vi "Read Sweep Rate.vi"(8 "error in (no error)":errorcluster, 11 "Power Supply in":refnum<class "Power Supply.lvclass">) -> (0 "error out":errorcluster, 2 "Field sweep rate":dbl[unit], 3 "Power Supply out":refnum<class "Power Supply.lvclass">)   [LabVIEW 2009, in "Power Supply.lvclass"]
uses:
  Power Supply.lvclass
  Power Supply.lvclass/Power Supply.ctl
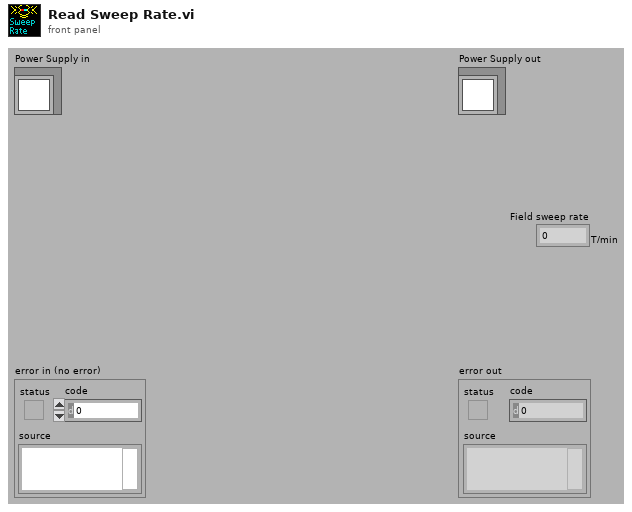
[diagram p1: front panel]
types:
  T1 = typedef "PSIO.ctl" = cluster{"Address":T2, "Version":enum16{"PS", "IPS"}}
  T2 = typedef "OxfordAddress.ctl" = cluster{"Com Port":i32, "ISOBUS Address":i32, "GPIB Address":i16, "Communication":enum16{"RS232", "ISOBUS", "GPIB", "Gateway"}}
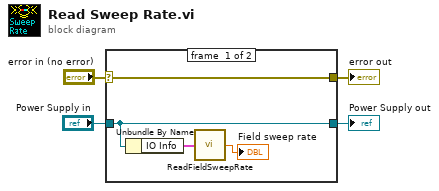
[diagram p0: block diagram]
diagram:
  n1 = case shown="No Error" "error in (no error)" {
    selector: "error in (no error)" -> [w6 w10]
    tunnel: "Power Supply in" -> [w5 w9]
    tunnel: [w6 w10] -> w2
    tunnel: [w5 w9] -> w1
    frame #0 {
      n2 = Unbundle By Name(w5) -> ("IO Info"=w7:T1)
      n3 = call "ReadFieldSweepRate.vi"("IO Info"=w7) -> ("Field sweep rate"=→"Field sweep rate":dbl[unit])  [unwired: 2 out]
    }
    frame #1 {
    }
  }
  "error out" <- w2
  "Power Supply out" <- w1
